vi "Calibrate Accelerometer.vi"() -> (3 "Output":dbl[][](array[numeric]))   [LabVIEW 2015]
uses:
  <vilib>/Analysis/baseanly.llb/Mean (DBL).vi
  <vilib>/Analysis/NI_AALBase.lvlib
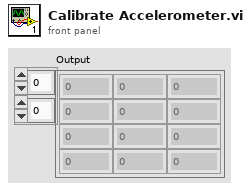
[diagram p1: front panel]
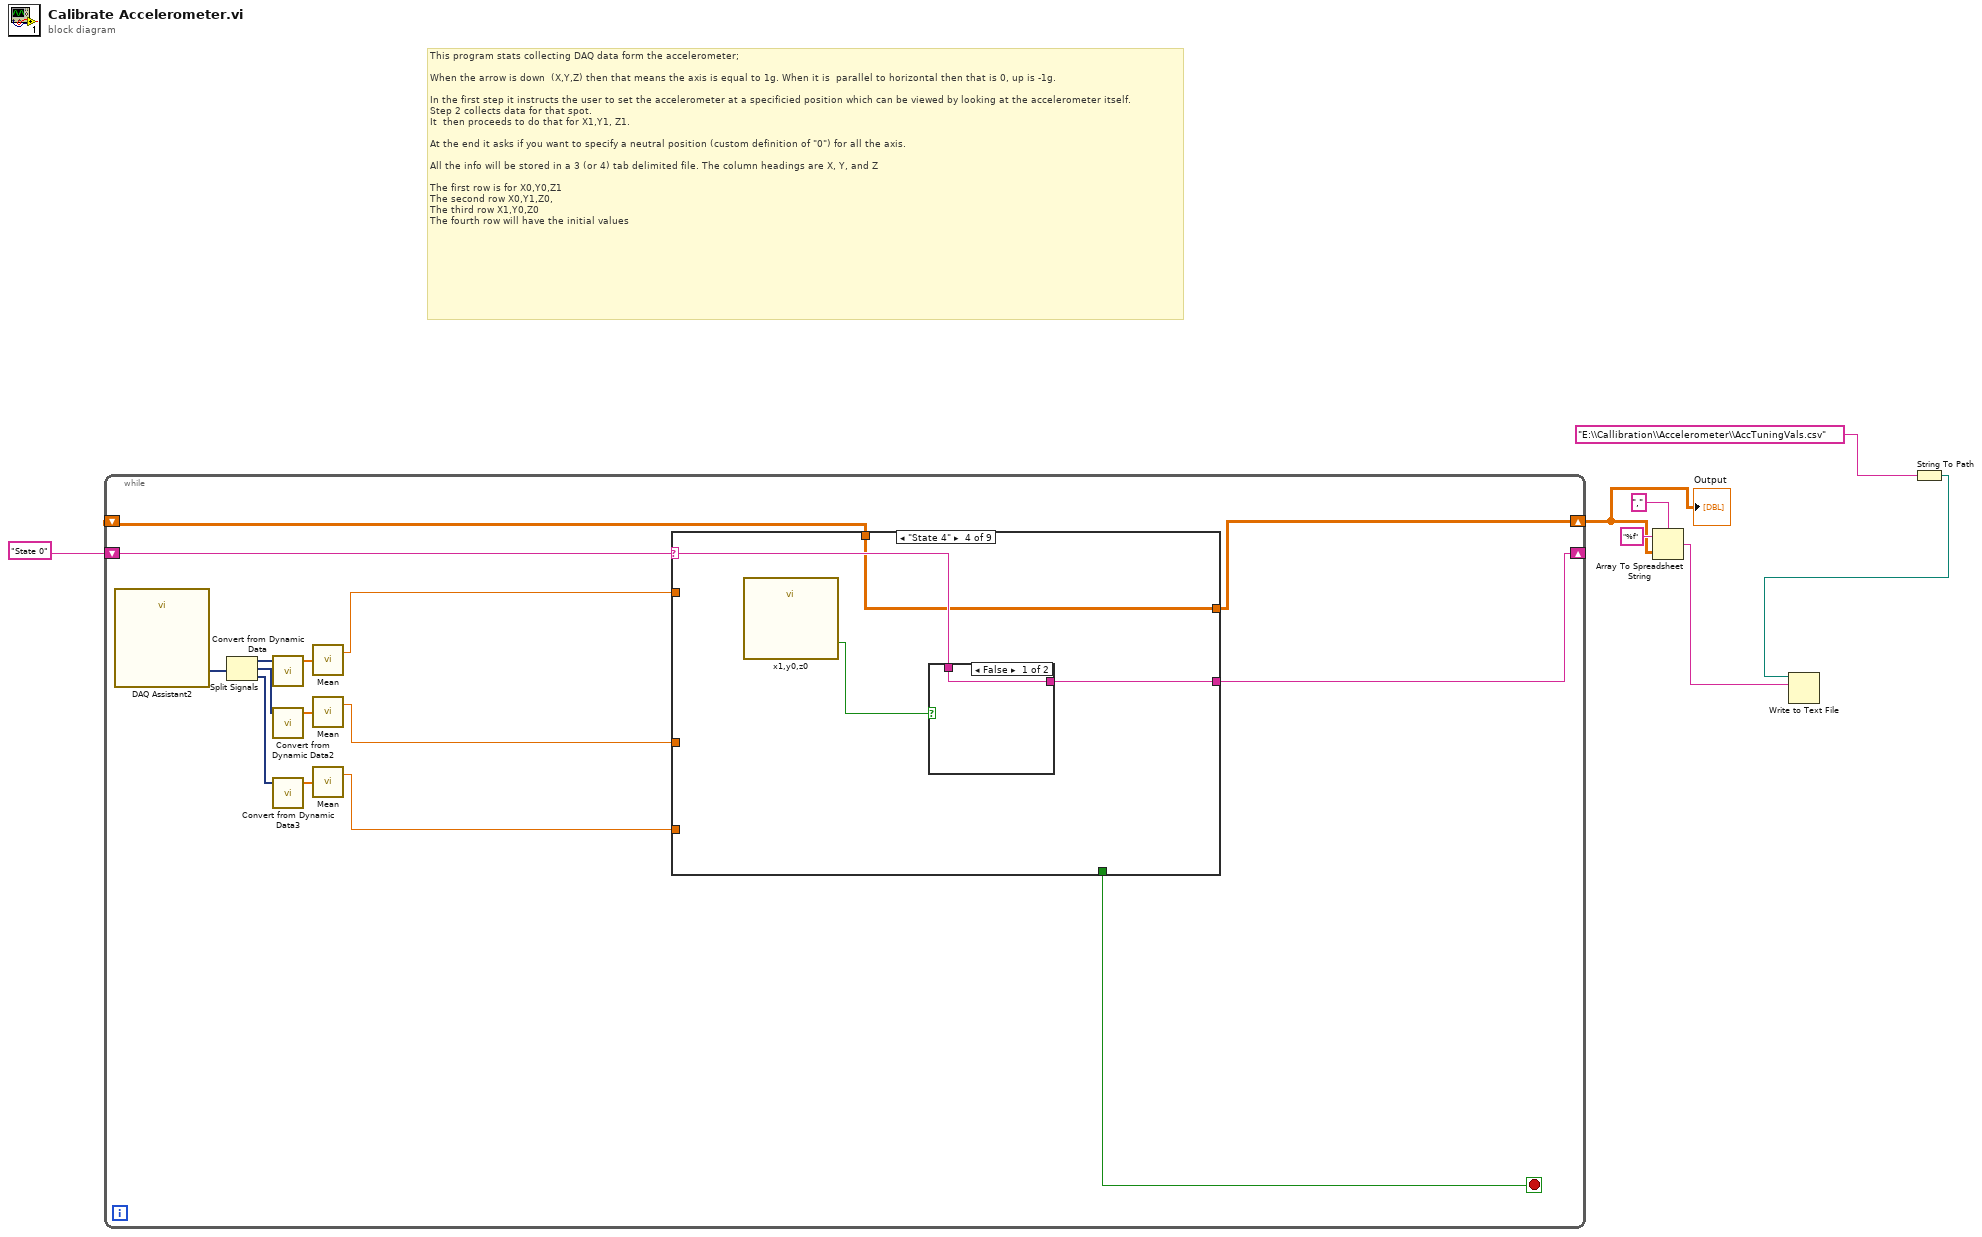
[diagram p0: block diagram]
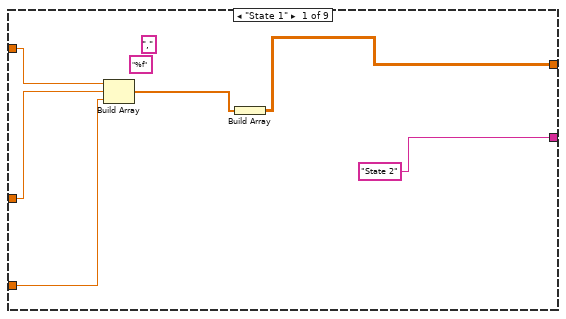
[diagram p2: hidden frame]
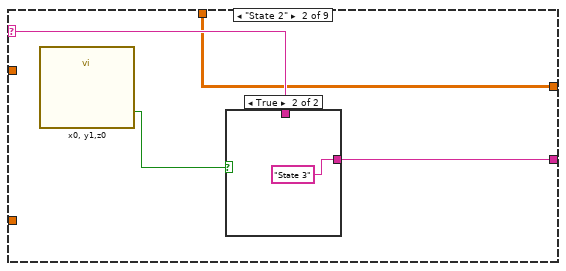
[diagram p3: hidden frame]
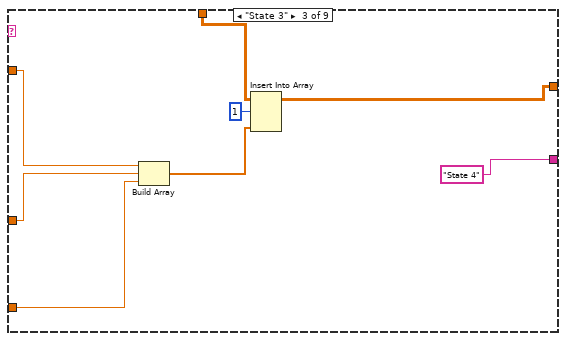
[diagram p5: hidden frame]
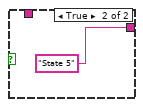
[diagram p6: hidden frame]
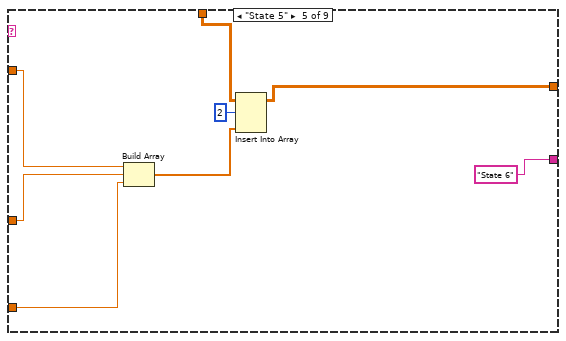
[diagram p7: hidden frame]
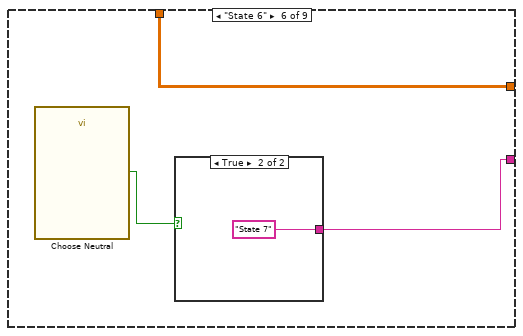
[diagram p8: hidden frame]
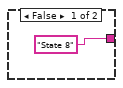
[diagram p9: hidden frame]
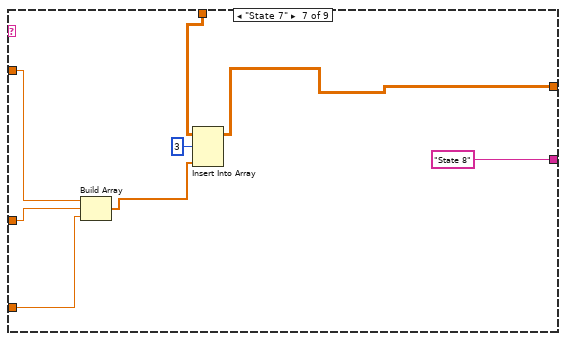
[diagram p10: hidden frame]
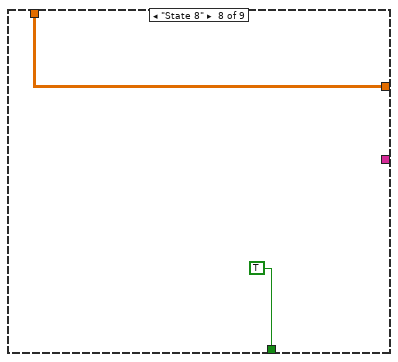
[diagram p11: hidden frame]
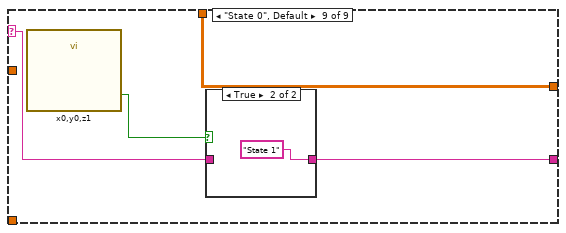
[diagram p12: hidden frame]
diagram:
  # "This program stats collecting DAQ data form the accelerometer;\n\nWhen the arrow is down  (X,Y,Z) then that means the axis is equal to 1g. When it is  parallel to horizontal then that is 0, up is -1g.\n\nIn the first step it instructs the user to set the accelerometer at a specificied position which can be viewed by looking at the accelerometer itself.\nStep 2 collects data for that spot. \nIt  then proceeds to do that for X1,Y1, Z1.\n\nAt the end it asks if you want to specify a neutral position (custom definition of \"0\") for all the axis. \n\nAll the info will be stored in a 3 (or 4) tab delimited file. The column headings are X, Y, and Z\n\nThe first row is for X0,Y0,Z1\nThe second row X0,Y1,Z0,\nThe third row X1,Y0,Z0\nThe fourth row will have the initial values"
  n1 = while {
    shift-right: [w12] -> _
    shift-left: "State 0" -> [w13]
    shift-right: [w10] -> w2
    shift-left: _ -> [w9]
    stop <- w11 stop-if-true
    n2 = call "DAQ Assistant2"() -> ("data"=w8:dynamicdata)  [unwired: 17 in, 2 out]
    n3 = Split Signals(w8) -> (w22:dynamicdata, w20:dynamicdata, w18:dynamicdata)  [unwired: 3 in]
    n4 = call "Convert from Dynamic Data"("Dynamic Data Type"=w22) -> ("Array"=w21:dbl[])  [unwired: 3 in]
    n5 = call "Convert from Dynamic Data2"("Dynamic Data Type"=w20) -> ("Array"=w19:dbl[])  [unwired: 3 in]
    n6 = call "Convert from Dynamic Data3"("Dynamic Data Type"=w18) -> ("Array"=w17:dbl[])  [unwired: 3 in]
    n7 = call-poly <vilib>:"Mean.vi"("X"=w21) -> ("mean"=w16:dbl)  [unwired: 1 out]
    n8 = call-poly <vilib>:"Mean.vi"("X"=w19) -> ("mean"=w15:dbl)  [unwired: 1 out]
    n9 = call-poly <vilib>:"Mean.vi"("X"=w17) -> ("mean"=w14:dbl)  [unwired: 1 out]
    n10 = case shown="\"State 4\"" w13 {
      selector: w13 -> [_ w30 _ w44 _ _ _ _ w73]
      tunnel: w16 -> [w28 _ w42 _ w56 _ w69 _ _]
      tunnel: w15 -> [w27 _ w41 _ w55 _ w68 _ _]
      tunnel: w14 -> [w26 _ w40 _ w54 _ w67 _ _]
      tunnel: ["State 2" w32 "State 4" w45 "State 6" w58 "State 8" _ w74] -> w12
      tunnel: [w23 w29 w38 w43 w52 w57 w65 w70 w72] -> w10
      tunnel: [_ _ _ _ _ _ _ TRUE _] -> w11
      tunnel: w9 -> [_ w29 w36 w43 w50 w57 w63 w70 w72]
      frame "State 1" {
        (unwired) "," ("delimiter (Tab)")
        (unwired) "%f" ("format string")
        n11 = Build Array(w28, w27, w26) -> (w24:dbl[])
        n12 = Build Array(w24) -> (w23:dbl[][])
      }
      frame "State 2" {
        n13 = call "x0, y1,z0"() -> ("OK"=w31:bool)  [unwired: 18 in, 1 out]
        n14 = case shown="True" w31 {
          tunnel: [w33 "State 3"] -> w32
          tunnel: w30 -> [w33 _]
          frame False {
          }
          frame True {
          }
        }
      }
      frame "State 3" {
        n15 = Build Array(w42, w41, w40) -> (w35:dbl[])
        n16 = Insert Into Array(array=w36, index (row)=1 ("index"), new element=w35) -> (w38:dbl[][])  [unwired: 1 in]
      }
      frame "State 4" {
        n17 = call "x1,y0,z0"() -> ("OK"=w46:bool)  [unwired: 18 in, 1 out]
        n18 = case shown="False" w46 {
          tunnel: [w47 "State 5"] -> w45
          tunnel: w44 -> [w47 _]
          frame False {
          }
          frame True {
          }
        }
      }
      frame "State 5" {
        n19 = Build Array(w56, w55, w54) -> (w49:dbl[])
        n20 = Insert Into Array(array=w50, index (row)=2 ("index"), new element=w49) -> (w52:dbl[][])  [unwired: 1 in]
      }
      frame "State 6" {
        n21 = call "Choose Neutral"() -> ("Yes"=w59:bool)  [unwired: 18 in, 1 out]
        n22 = case shown="True" w59 {
          tunnel: ["State 8" "State 7"] -> w58
          frame False {
          }
          frame True {
          }
        }
      }
      frame "State 7" {
        n23 = Build Array(w69, w68, w67) -> (w62:dbl[])
        n24 = Insert Into Array(array=w63, index (row)=3 ("index"), new element=w62) -> (w65:dbl[][])  [unwired: 1 in]
      }
      frame "State 8" {
      }
      frame "State 0", Default {
        n25 = call "x0,y0,z1"() -> ("OK"=w75:bool)  [unwired: 18 in, 1 out]
        n26 = case shown="True" w75 {
          tunnel: [w76 "State 1"] -> w74
          tunnel: w73 -> [w76 _]
          frame False {
          }
          frame True {
          }
        }
      }
    }
  }
  "Output" <- w2
  n27 = Array To Spreadsheet String(delimiter (Tab)=",", array=w2, 3:"%f" ("format string")) -> (spreadsheet string=w3:string)
  n28 = String To Path(string="E:\\Callibration\\Accelerometer\\AccTuningVals.csv") -> (path=w6:path)
  n29 = Write to Text File(file (use dialog)=w6, text=w3) -> ()  [unwired: 2 in, 3 out]
